vi "Simple Shared Memory.vi"() -> ()   [LabVIEW 2013]
uses:
  Source/Shared Memory/Classes/Shared Memory/Public/Controls/file mode.ctl
  Source/Shared Memory/Pointer Operations/Write String.vi
  Source/Shared Memory/Pointer Operations/Read String.vi
  Source/Shared Memory/Pointer Operations/Write Scalar I32.vi
  Source/Shared Memory/Pointer Operations/Read Scalar I32.vi
  Source/Shared Memory/Pointer Operations/Write Scalar DBL.vi
  Source/Shared Memory/Pointer Operations/Read Scalar DBL.vi
  Source/Shared Memory/Pointer Operations/Write Scalar Boolean.vi
  Source/Shared Memory/Pointer Operations/Read Scalar Boolean.vi
  Source/Shared Memory/Shared Memory.lvlib
  Source/Shared Memory/Classes/Shared Memory/Shared Memory.lvclass
panel:
  in  "String Write":string
  out "String Read":string
  out "Boolean Read":bool
  out "Double Read":dbl
  out "Integer Read":i32
  in  "Integer Write":i32
  in  "Double Write":dbl
  in  "Boolean Write":bool
  in  "stop":bool
  # "NOTE: The provided C application hasn't been updated to read the string that LabVIEW writes to memory."
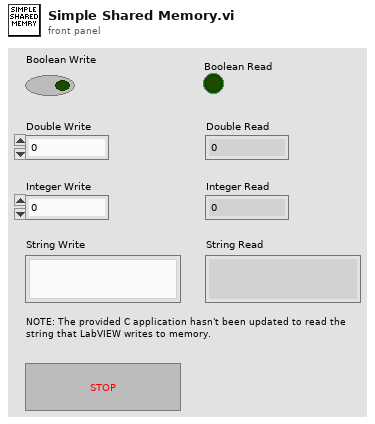
[diagram p1: front panel]
types:
  T1 = typedef "Linux RT IPC.lvlib/Shared Memory.lvlib/file mode.ctl" = enum16{"open", "create/replace"}
  T2 = typedef "Linux RT IPC.lvlib/Shared Memory.lvlib/Shared Memory.lvclass/reference.ctl" = refnum<data-value>
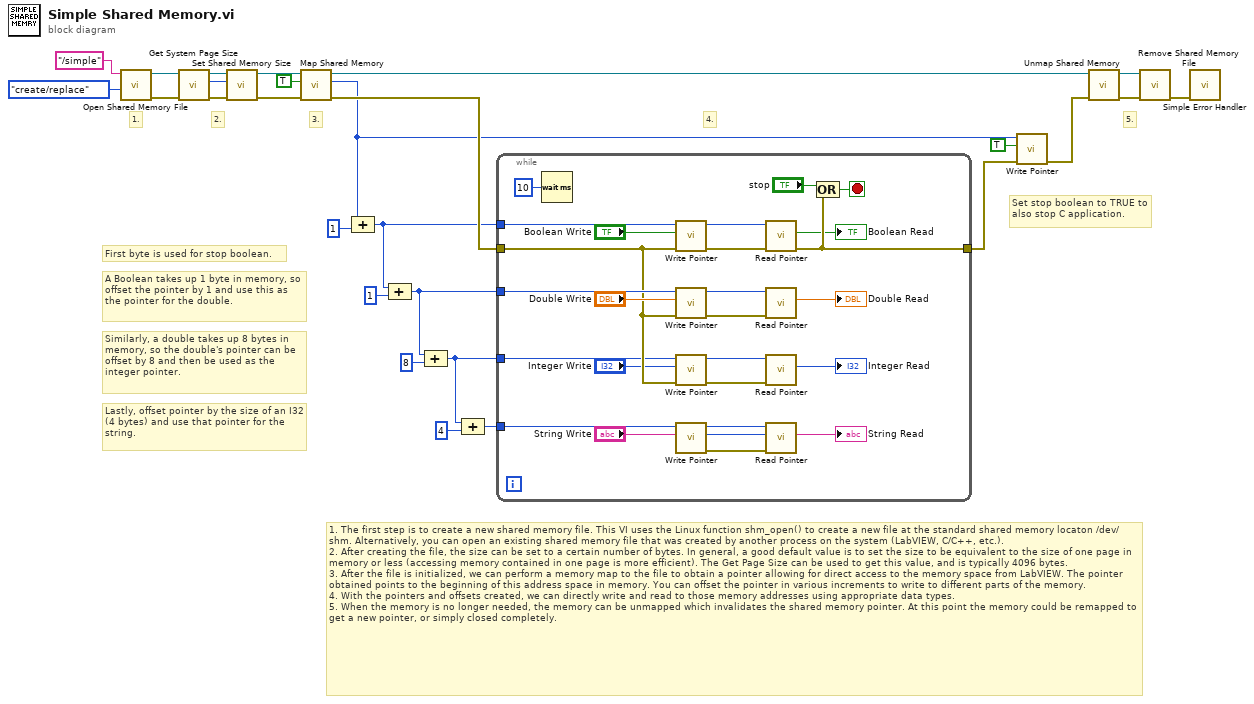
[diagram p0: block diagram]
diagram:
  # "Lastly, offset pointer by the size of an I32 (4 bytes) and use that pointer for the string."
  # "First byte is used for stop boolean."
  # "Set stop boolean to TRUE to also stop C application."
  # "4."
  # "Similarly, a double takes up 8 bytes in memory, so the double's pointer can be offset by 8 and then be used as the integer pointer."
  # "A Boolean takes up 1 byte in memory, so offset the pointer by 1 and use this as the pointer for the double."
  # "1. The first step is to create a new shared memory file. This VI uses the Linux function shm_open() to create a new file at the standard shared memory locaton /dev/shm. Alternatively, you can open an existing shared memory file that was created by another process on the system (LabVIEW, C/C++, etc.).\n2. After creating the file, the size can be set to a certain number of bytes. In general, a good default value is to set the size to be equivalent to the size of one page in memory or less (accessing memory contained in one page is more efficient). The Get Page Size can be used to get this value, and is typically 4096 bytes.\n3. After the file is initialized, we can perform a memory map to the file to obtain a pointer allowing for direct access to the memory space from LabVIEW. The pointer obtained points to the beginning of this address space in memory. You can offset the pointer in various increments to write to different parts of the memory.\n4. With the pointers and offsets created, we can directly write and read to those memory addresses using appropriate data types.\n5. When the memory is no longer needed, the memory can be unmapped which invalidates the shared memory pointer. At this point the memory could be remapped to get a new pointer, or simply closed completely."
  # "5."
  # "3."
  # "2."
  # "1."
  n1 = call "Open Shared Memory File.vi"("file mode (open)"=file_mode."create/replace" ("file mode (default: open)"), "shared memory name"="/simple") -> ("error out"=w26:errorcluster, "shared memory out"=w27:T2)  [unwired: 8 in]
  n2 = call "Get System Page Size.vi"("error in (no error)"=w26, "shared memory in"=w27) -> ("error out"=w23:errorcluster, "page size (bytes)"=w25:u32, "shared memory out"=w24:T2)  [unwired: 7 in]
  n3 = call "Set Shared Memory Size.vi"("error in (no error)"=w23, "size (bytes)"=w25, "shared memory in"=w24) -> ("error out"=w21:errorcluster, "shared memory out"=w22:T2)  [unwired: 7 in]
  n4 = call "Map Shared Memory.vi"("error in (no error)"=w21, "close file descriptor on success? (F)"=TRUE ("auto-close file descriptor on success? (T)"), "shared memory in"=w22) -> ("error out"=w14:errorcluster, "pointer to shared memory"=w7:u64, "shared memory out"=w10:T2)  [unwired: 6 in]
  n5 = Compound Arithmetic op=ADD(w7, u64 1 ("value")) -> (w8:u64)
  n6 = Compound Arithmetic op=ADD(w8, u64 1 ("value")) -> (w17:u64)
  n7 = Compound Arithmetic op=ADD(w17, u64 8 ("value")) -> (w1:u64)
  n8 = Compound Arithmetic op=ADD(w1, u64 4 ("value")) -> (w2:u64)
  n9 = while {
    tunnel: w8 -> [w50]
    tunnel: w17 -> [w44]
    tunnel: w1 -> [w40]
    tunnel: w14 -> [w42]
    tunnel: [w47] -> w6
    tunnel: w2 -> [w28]
    stop <- w51 stop-if-true
    n10 = Wait (ms)(milliseconds to wait=u32 10) -> ()  [unwired: 1 out]
    n11 = call-poly "Write Pointer.vi"("error in (no error)"=w42, "value"="Boolean Write", "pointer in"=w50) -> ("error out"=w48:errorcluster, "pointer out"=w49:u64)  [unwired: 7 in]
    n12 = call-poly "Write Pointer.vi"("error in (no error)"=w42, "value"="Double Write", "pointer in"=w44) -> ("error out"=w37:errorcluster, "pointer out"=w39:u64)  [unwired: 7 in]
    n13 = call-poly "Write Pointer.vi"("error in (no error)"=w42, "value"="Integer Write", "pointer in"=w40) -> ("error out"=w36:errorcluster, "pointer out"=w38:u64)  [unwired: 7 in]
    n14 = call-poly "Write Pointer.vi"("string in"="String Write", "pointer in"=w28) -> ("error out"=w31:errorcluster, "bytes written"=w33:i64, "pointer out"=w32:u64)  [unwired: 6 in, 1 out]
    n15 = call-poly "Read Pointer.vi"("error in (no error)"=w48, "pointer in"=w49) -> ("error out"=w47:errorcluster, "value"=→"Boolean Read":bool)  [unwired: 7 in, 1 out]
    n16 = call-poly "Read Pointer.vi"("error in (no error)"=w37, "pointer in"=w39) -> ("value"=→"Double Read":dbl)  [unwired: 7 in, 2 out]
    n17 = call-poly "Read Pointer.vi"("error in (no error)"=w36, "pointer in"=w38) -> ("value"=→"Integer Read":i32)  [unwired: 7 in, 2 out]
    n18 = call-poly "Read Pointer.vi"("error in (no error)"=w31, "bytes to read"=w33, "pointer in"=w32) -> ("string out"=→"String Read":string)  [unwired: 6 in, 2 out]
    n19 = Compound Arithmetic op=OR("stop", w47) -> (w51:bool)
  }
  n20 = call-poly "Write Pointer.vi"("error in (no error)"=w6, "value"=TRUE, "pointer in"=w7) -> ("error out"=w5:errorcluster)  [unwired: 7 in, 1 out]
  n21 = call "Unmap Shared Memory.vi"("error in (no error)"=w5, "shared memory in"=w10) -> ("error out"=w13:errorcluster, "shared memory out"=w12:T2)  [unwired: 8 in]
  n22 = call "Remove Shared Memory File.vi"("error in (no error)"=w13, "shared memory in"=w12) -> ("error out"=w11:errorcluster)  [unwired: 8 in, 1 out]
  n23 = call <vilib>:"Simple Error Handler.vi"("error in (no error)"=w11) -> ()  [unwired: 4 in, 5 out]
